vi "HGF_DSCCommand.appendData2Variant.vi"(0 "initData":variant, 2 "SV":refnum<k21>, 3 "typeDescriptor":string, 5 "error in (no error)":errorcluster, 6 "initValue":string) -> (14 "dup initData":variant, 19 "error out":errorcluster)   [LabVIEW 2012, in "HGF_DSC.lvlib" / "HGF_DSCCommand.lvclass"]
uses:
  HGF_DSCCommand.lvclass
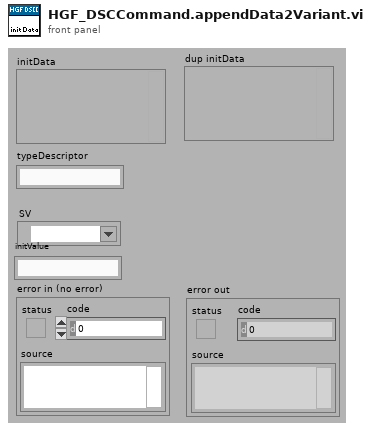
[diagram p1: front panel]
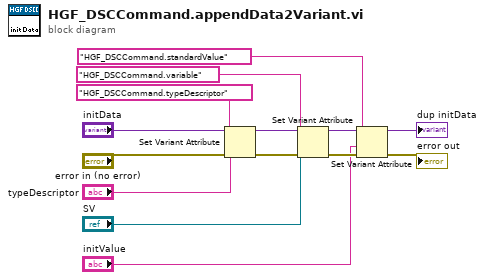
[diagram p0: block diagram]
diagram:
  n1 = Set Variant Attribute(Variant="initData", name="HGF_DSCCommand.typeDescriptor", value="typeDescriptor", error in="error in (no error)") -> (Variant out=w12:variant, error out=w14:errorcluster)  [unwired: 1 out]
  n2 = Set Variant Attribute(Variant=w12, name="HGF_DSCCommand.variable", value="SV", error in=w14) -> (Variant out=w4:variant, error out=w6:errorcluster)  [unwired: 1 out]
  n3 = Set Variant Attribute(Variant=w4, name="HGF_DSCCommand.standardValue", value="initValue", error in=w6) -> (Variant out=→"dup initData":variant, error out=→"error out":errorcluster)  [unwired: 1 out]
